vi "changefilename.vi"(2 "suffix":string, 3 "path in":path) -> (0 "orig filetype":string, 1 "path out":path)   [LabVIEW 2009]
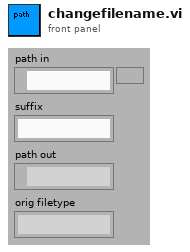
[diagram p1: front panel]
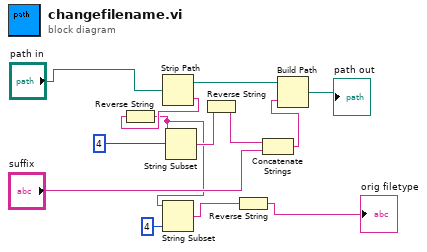
[diagram p0: block diagram]
diagram:
  n1 = Strip Path(path="path in") -> (stripped path=w13:path, name=w12:string)
  n2 = Reverse String(1:w12) -> (0:w4:string)
  n3 = String Subset(string=w4, length (rest)=4 ("Länge (Rest)")) -> (substring=w2:string)  [unwired: 1 in]
  n4 = String Subset(string=w4, offset (0)=4 ("Offset (0)")) -> (substring=w7:string)  [unwired: 1 in]
  n5 = Reverse String(1:w7) -> (0:w8:string)
  n6 = Reverse String(1:w2) -> (0:→"orig filetype":string)
  n7 = Concatenate Strings(w8, "suffix") -> (w10:string)
  n8 = Build Path(base path=w13, name or relative path=w10) -> (appended path=→"path out":path)
